vi "Set Channel Settings.vi"(8 "error in (no error)":errorcluster, 10 "settings":T1, 11 "channel in":T2={"string offset"=0, "name"="Channel", "units"="V", "engine data type"=enum."DBL", "string data type"=enum."DBL", "settings"=[]} {"string offset" format="%d bytes"}) -> (0 "error out":errorcluster, 3 "channel out":T2={"string offset"=0, "name"="Channel", "units"="V", "engine data type"=enum."DBL", "string data type"=enum."DBL", "settings"=[]} {"string offset" format="%d bytes"})   [LabVIEW 2017, in "DSF Core.lvlib" / "Configuration Session.lvclass"]
uses:
  Configuration Session.lvclass
  Typedefs/DSF Engine Channel Configuration.ctl
  Typedefs/DSF Data Type.ctl
  Typedefs/DSF Settings Info.ctl
  DSF Core.lvlib
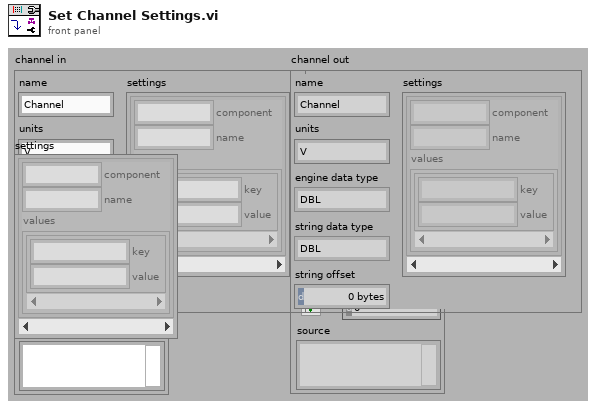
[diagram p1: front panel]
types:
  T1 = typedef "DSF Core.lvlib/DSF Settings Info.ctl" = cluster{"component":string, "name":string, "values":cluster{"key":string, "value":string}[]}[]
  T2 = typedef "DSF Core.lvlib/DSF Engine Channel Configuration.ctl" = cluster{"string offset":u64, "name":string, "units":string, "engine data type":T3, "string data type":T3, "settings":T1}
  T3 = typedef "DSF Core.lvlib/DSF Data Type.ctl" = enum8{"Bool", "SGL", "DBL", "I8", "I16", "I32", "I64", "U8", "U16", "U32", "U64"}
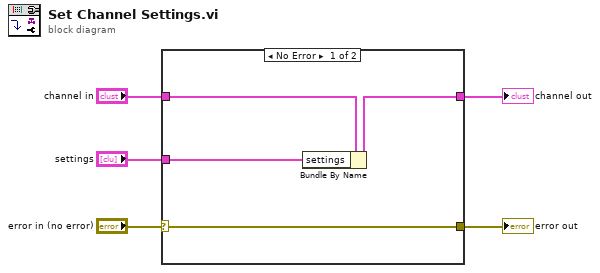
[diagram p0: block diagram]
diagram:
  n1 = case shown="No Error" "error in (no error)" {
    selector: "error in (no error)" -> [w7 w11]
    tunnel: [w7 w11] -> w5
    tunnel: [w8 w10] -> w2
    tunnel: "channel in" -> [w9 w10]
    tunnel: "settings" -> [w6 _]
    frame No Error {
      n2 = Bundle By Name(cluster=w9, "settings"=w6) -> (w8:T2)
    }
    frame Error {
    }
  }
  "error out" <- w5
  "channel out" <- w2
